vi "Main.vi"() -> ()   [LabVIEW 2014, in "Chart Module.lvlib"]
uses:
  Chart Module.lvlib
  Module Data--cluster.ctl
  Limits Argument--cluster.ctl
  <vilib>/Delacor/Delacor QMH/Libraries/Message Queue_class/Delacor_lib_QMH_Message Queue.lvclass/Delacor_lib_QMH_Message Queue.ctl
  Send Value Argument--cluster.ctl
  Show Panel Argument--cluster.ctl
  Position--enum.ctl
  Stop Argument--cluster.ctl
  <vilib>/Delacor/Delacor QMH/Libraries/Message Queue_class/Delacor_lib_QMH_Enqueue Message (Single).vi
  <vilib>/Delacor/Delacor QMH/Libraries/Message Queue_class/Delacor_lib_QMH_Message Queue.lvclass
panel:
  in  "Title":bool
  out "Chart":T1(graph)
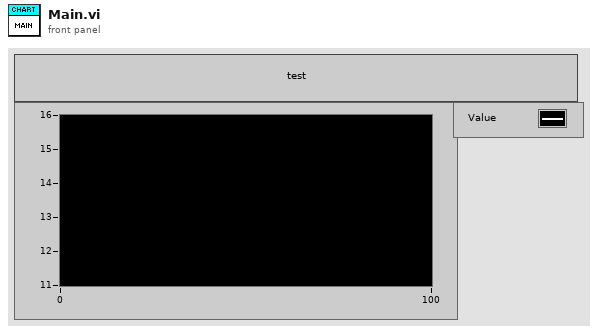
[diagram p1: front panel]
types:
  T1 = cluster{"Value":dbl, "HighLim":dbl, "LowLim":dbl}
  T2 = typedef "Chart Module.lvlib/Request Events--cluster.ctl" = cluster{"Stop Module":refnum<user-event>, "Show Panel":refnum<user-event>, "Hide Panel":refnum<user-event>, "Update Limits":refnum<user-event>, "Send Value":refnum<user-event>, "Clear Chart":refnum<user-event>, "Show Block Diagram":refnum<user-event>}
  T3 = typedef "Chart Module.lvlib/Module Data--cluster.ctl" = cluster{"Status":string, "Limits ":T4}
  T4 = typedef "Chart Module.lvlib/Limits Argument--cluster.ctl" = cluster{"Enabled?":bool, "HighLim":dbl, "LowLim":dbl}
  T5 = typedef "Chart Module.lvlib/Stop Argument--cluster.ctl" = cluster{"Origin":string, "Exit via Stop Module Req?":bool}
  T6 = typedef "Chart Module.lvlib/Show Panel Argument--cluster.ctl" = cluster{"Show Chart?":bool, "Chart Title":string, "Window Position":T7}
  T7 = typedef "Chart Module.lvlib/Position--enum.ctl" = enum16{"Upper-Left", "Upper-Center", "Upper-Right", "Center-left", "Center", "Center-Right", "Bottom-Left", "Bottom-Center", "Bottom-Right", ""}
  T8 = typedef "Chart Module.lvlib/Send Value Argument--cluster.ctl" = cluster{"Value":dbl}
  T9 = cluster{"Shift":bool, "Ctrl":bool, "Alt":bool, "Cmd":bool, "Opt":bool}
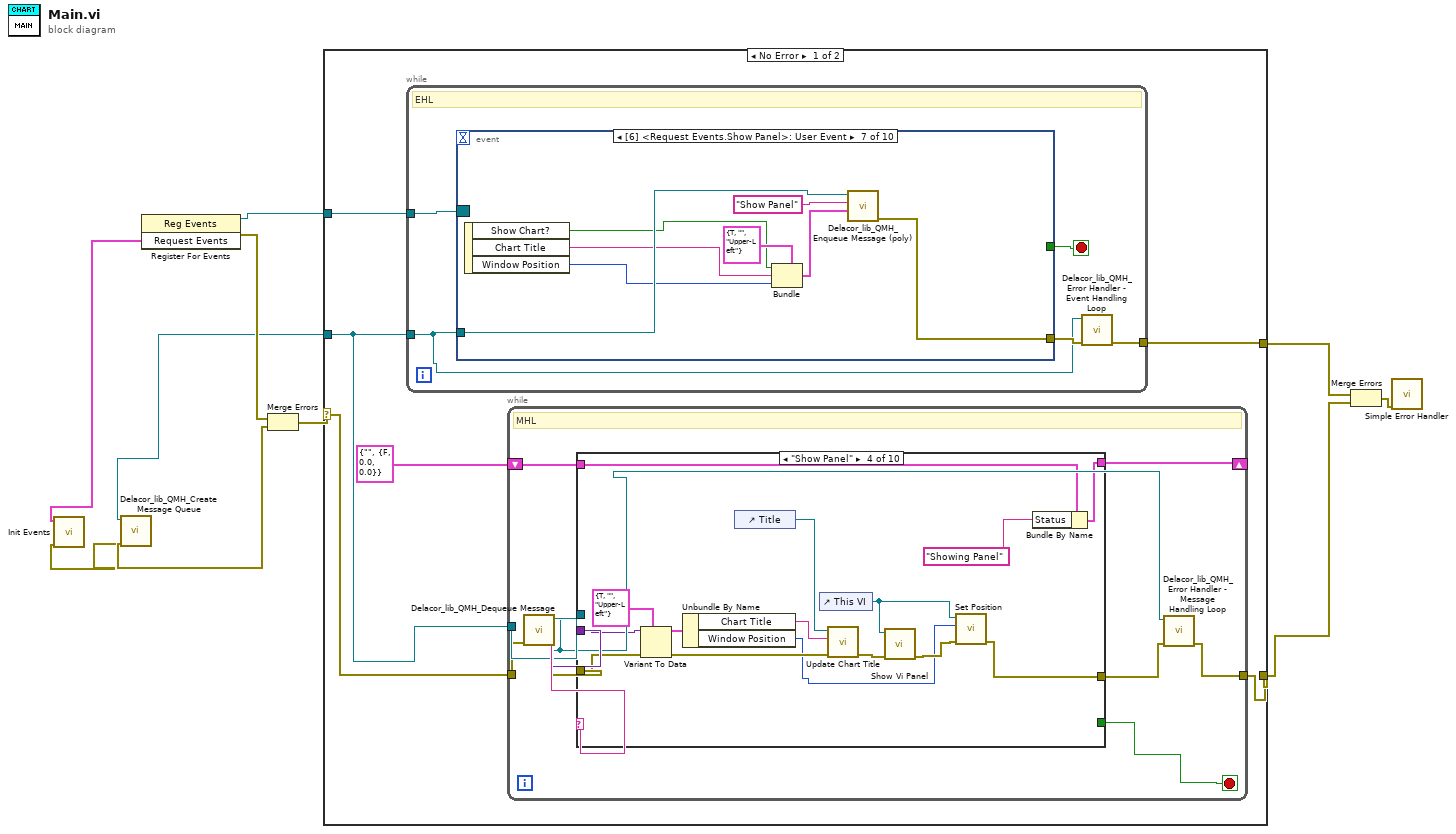
[diagram p0: block diagram]
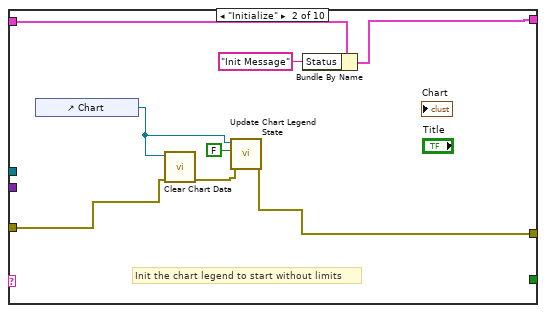
[diagram p3: hidden frame]
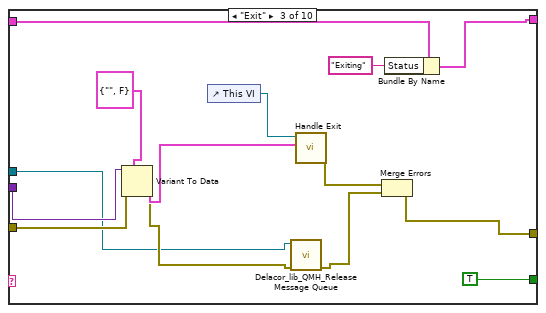
[diagram p4: hidden frame]
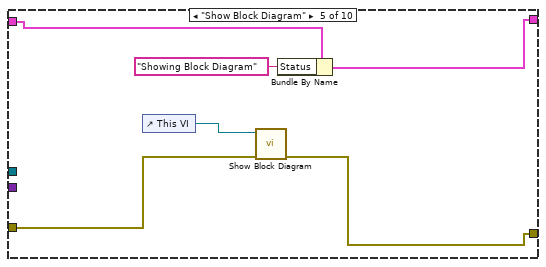
[diagram p5: hidden frame]
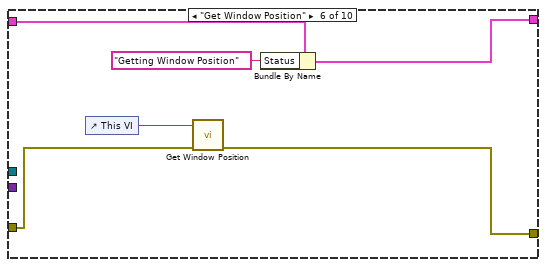
[diagram p6: hidden frame]
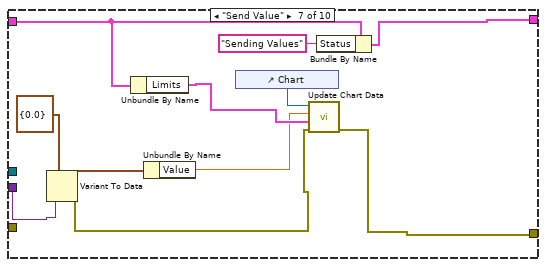
[diagram p7: hidden frame]
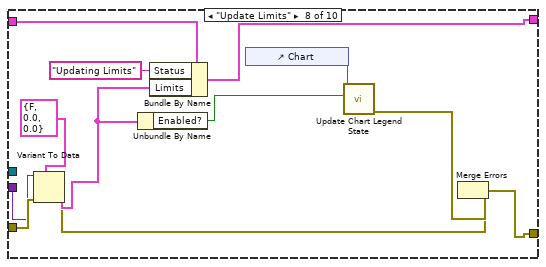
[diagram p8: hidden frame]
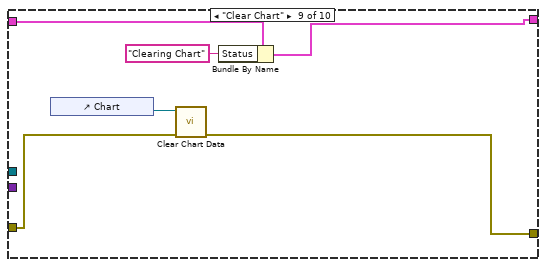
[diagram p9: hidden frame]
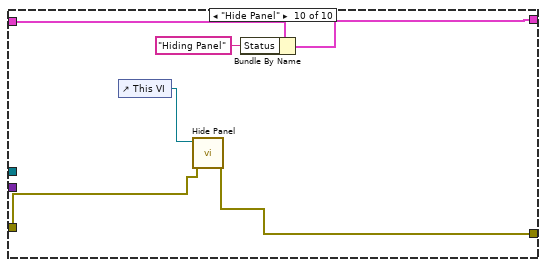
[diagram p10: hidden frame]
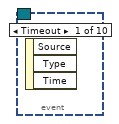
[diagram p11: hidden frame]
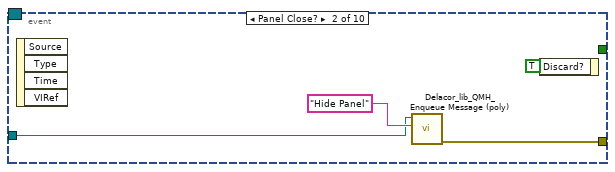
[diagram p12: hidden frame]
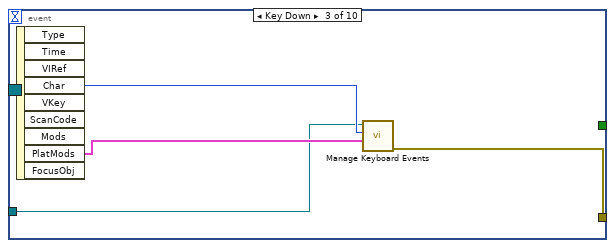
[diagram p13: hidden frame]
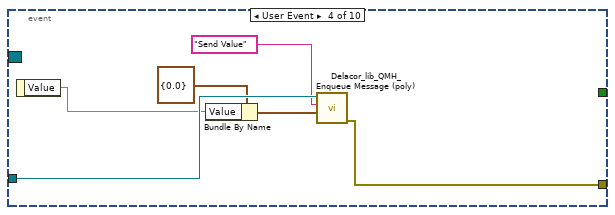
[diagram p14: hidden frame]
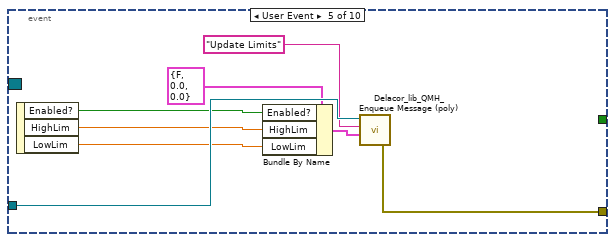
[diagram p15: hidden frame]
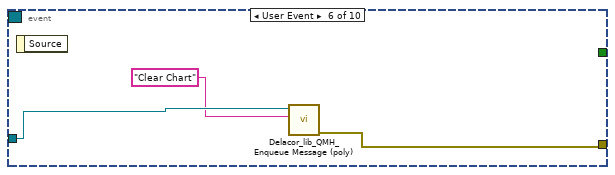
[diagram p16: hidden frame]
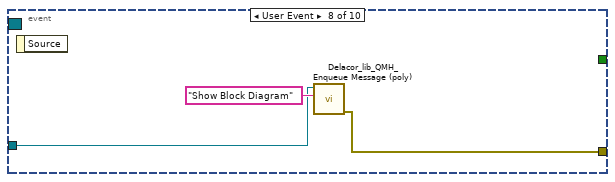
[diagram p17: hidden frame]
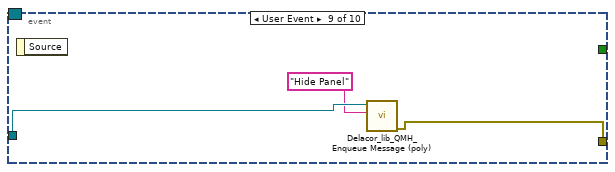
[diagram p18: hidden frame]
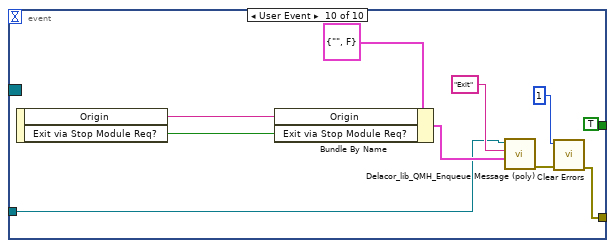
[diagram p19: hidden frame]
diagram:
  n1 = call "Init Events.vi"() -> ("error out"=w5:errorcluster, "Request Events"=w6:T2)  [unwired: 10 in]
  n2 = call <vilib>:"Delacor_lib_QMH_Create Message Queue.vi"("error in"=w5) -> ("error out"=w7:errorcluster, "Message Queue"=w4:refnum<class "Delacor_lib_QMH_Message Queue.lvclass">)  [unwired: 9 in]
  n3 = register-events(w6) -> (reference out=w8:refnum<event-registration>, error out=w9:errorcluster)  [unwired: 2 in]
  n4 = Merge Errors(w9, w7) -> (w10:errorcluster)
  n5 = case shown="No Error" w10 {
    selector: w10 -> [w11 _]
    tunnel: w8 -> [w16 _]
    tunnel: w4 -> [w15 _]
    tunnel: [w14 _] -> w3
    tunnel: [w13 _] -> w2
    frame No Error {
      n6 = while {
        tunnel: w16 -> [w118]
        tunnel: w15 -> [w114]
        tunnel: [w116] -> w14
        stop <- w115 stop-if-true
        # "EHL"
        n7 = event shown="[6] <Request Events.Show Panel>: User Event" {
          selector: w118 -> [_ _ _ _ _ _ _ _ _ _]
          dyn-events: _ -> [_ _ _ _ _ _ _ _ _ _]
          timeout: _ -> [_ _ _ _ _ _ _ _ _ _]
          tunnel: w114 -> [_ w121 w124 w132 w140 w143 w151 w152 w157 w162]
          tunnel: [_ w120 w123 w130 w133 w141 w149 w153 w155 w159] -> w117
          tunnel: [_ _ _ _ _ _ _ _ _ TRUE] -> w115
          event Timeout {
            n8 = event-data() -> ()  [unwired: 1 in, 3 out]
          }
          event Panel Close? {
            n9 = event-data() -> ()  [unwired: 1 in, 4 out]
            n10 = call-poly <vilib>:"Delacor_lib_QMH_Enqueue Message (poly).vi"("Message"="Hide Panel", "Message Queue in"=w121) -> ("error out"=w120:errorcluster)  [unwired: 8 in, 1 out]
            n11 = event-data("Discard?"=TRUE) -> ()  [unwired: 1 in, 1 out]
          }
          event Key Down {
            n12 = event-data() -> ("Char"=w125:i16, "PlatMods"=w126:T9)  [unwired: 1 in, 7 out]
            n13 = call "Manage Keyboard Events.vi"("PlatMods"=w126, "Char"=w125, "Delacor_lib_QMH_Message Queue in"=w124) -> ("error out"=w123:errorcluster)  [unwired: 8 in]
          }
          event User Event {
            n14 = event-data() -> ("Value"=w128:dbl)  [unwired: 1 in]
            n15 = Bundle By Name(cluster=T8 {"Value"=0.0} ("Send Value Argument"), "Value"=w128) -> (w127:T8)
            n16 = call-poly <vilib>:"Delacor_lib_QMH_Enqueue Message (poly).vi"("Message Data"=w127, "Message"="Send Value", "Message Queue in"=w132) -> ("error out"=w130:errorcluster)  [unwired: 7 in, 1 out]
          }
          event User Event {
            n17 = event-data() -> ("Enabled?"=w135:bool, "HighLim"=w136:dbl, "LowLim"=w137:dbl)  [unwired: 1 in]
            n18 = Bundle By Name(cluster=T4 {"Enabled?"=FALSE, "HighLim"=0.0, "LowLim"=0.0} ("Limits Argument"), "Enabled?"=w135, "HighLim"=w136, "LowLim"=w137) -> (w134:T4)
            n19 = call-poly <vilib>:"Delacor_lib_QMH_Enqueue Message (poly).vi"("Message Data"=w134, "Message"="Update Limits", "Message Queue in"=w140) -> ("error out"=w133:errorcluster)  [unwired: 7 in, 1 out]
          }
          event User Event {
            n20 = event-data() -> ()  [unwired: 1 in, 1 out]
            n21 = call-poly <vilib>:"Delacor_lib_QMH_Enqueue Message (poly).vi"("Message"="Clear Chart", "Message Queue in"=w143) -> ("error out"=w141:errorcluster)  [unwired: 8 in, 1 out]
          }
          event User Event {
            n22 = event-data() -> ("Show Chart?"=w147:bool, "Chart Title"=w146:string, "Window Position"=w144:T7)  [unwired: 1 in]
            n23 = Bundle(cluster=T6 {"Show Chart?"=TRUE, "Chart Title"="", "Window Position"=enum."Upper-Left"} ("Show Panel Argument"), "Show Chart?"=w147, "Chart Title"=w146, "Window Position"=w144) -> (w145:T6)
            n24 = call-poly <vilib>:"Delacor_lib_QMH_Enqueue Message (poly).vi"("Message Data"=w145, "Message"="Show Panel", "Message Queue in"=w151) -> ("error out"=w149:errorcluster)  [unwired: 7 in, 1 out]
          }
          event User Event {
            n25 = event-data() -> ()  [unwired: 1 in, 1 out]
            n26 = call-poly <vilib>:"Delacor_lib_QMH_Enqueue Message (poly).vi"("Message"="Show Block Diagram", "Message Queue in"=w152) -> ("error out"=w153:errorcluster)  [unwired: 8 in, 1 out]
          }
          event User Event {
            n27 = event-data() -> ()  [unwired: 1 in, 1 out]
            n28 = call-poly <vilib>:"Delacor_lib_QMH_Enqueue Message (poly).vi"("Message"="Hide Panel", "Message Queue in"=w157) -> ("error out"=w155:errorcluster)  [unwired: 8 in, 1 out]
          }
          event User Event {
            n29 = event-data() -> ("Origin"=w167:string, "Exit via Stop Module Req?"=w166:bool)  [unwired: 1 in]
            n30 = Bundle By Name(cluster=T5 {"Origin"="", "Exit via Stop Module Req?"=FALSE} ("Stop Argument"), "Origin"=w167, "Exit via Stop Module Req?"=w166) -> (w164:T5)
            n31 = call-poly <vilib>:"Delacor_lib_QMH_Enqueue Message (poly).vi"("Message Data"=w164, "Message"="Exit", "Message Queue in"=w162) -> ("error out"=w160:errorcluster)  [unwired: 7 in, 1 out]
            n32 = call <vilib>:"Clear Errors.vi"("error in (no error)"=w160, "specific error code to clear (0: all)"=1) -> ("error out"=w159:errorcluster)  [unwired: 4 in, 1 out]
          }
        }
        n33 = call-dynamic "Delacor_lib_QMH_Error Handler - Event Handling Loop.vi"("error in"=w117, "Message Queue in"=w114) -> ("dup error in"=w116:errorcluster)  [unwired: 8 in, 1 out]
      }
      n34 = while {
        tunnel: w15 -> [w22]
        tunnel: [w24] -> w13
        shift-right: [w19] -> _
        shift-left: T3 {"Status"="", "Limits "={"Enabled?"=FALSE, "HighLim"=0.0, "LowLim"=0.0}} ("Module Data") -> [w20]
        tunnel: w11 -> [w18]
        stop <- w21 stop-if-true
        # "MHL"
        n35 = call-dynamic "Delacor_lib_QMH_Dequeue Message.vi"("error in"=w18, "Message Queue in"=w22) -> ("error out"=w25:errorcluster, "Message Data"=w26:variant, "Message"=w27:string, "Message Queue out"=w17:refnum<class "Delacor_lib_QMH_Message Queue.lvclass">)  [unwired: 6 in]
        n36 = case shown="\"Show Panel\"" w27 {
          tunnel: w17 -> [_ _ w43 _ _ _ _ _ _ _]
          tunnel: w26 -> [_ _ w50 w61 _ _ w89 w100 _ _]
          tunnel: w25 -> [w29 w34 w49 w63 w71 w75 _ w101 w107 w112]
          tunnel: [w29 w32 w44 w55 w70 w74 w81 w93 w106 w111] -> w23
          tunnel: [_ _ TRUE _ _ _ _ _ _ _] -> w21
          tunnel: w20 -> [w28 w37 w40 w66 w69 w77 w86 w98 w105 w110]
          tunnel: [w28 w36 w39 w65 w68 w78 w85 w97 w104 w109] -> w19
          frame "Def", Default {
          }
          frame "Initialize" {
            # "Init the chart legend to start without limits"
            n37 = control-ref of="Chart"() -> (w31:refnum<vi>)
            n38 = call "Clear Chart Data.vi"("error in (no error)"=w34, "WaveformChart in"=w31) -> ("error out"=w33:errorcluster)  [unwired: 9 in]
            n39 = call "Update Chart Legend State.vi"("error in"=w33, "Enabled?"=FALSE, "WaveformChart in"=w31) -> ("error out"=w32:errorcluster)  [unwired: 8 in]
            n40 = Bundle By Name(cluster=w37, "Status"="Init Message") -> (w36:T3)
          }
          frame "Exit" {
            n41 = Variant To Data(error in=w49, type=T5 {"Origin"="", "Exit via Stop Module Req?"=FALSE} ("Stop Argument"), Variant=w50) -> (data=w48:T5, error out=w47:errorcluster)
            n42 = control-ref of="This VI"() -> (w41:refnum<vi>)
            n43 = call-dynamic "Delacor_lib_QMH_Release Message Queue.vi"("error in"=w47, "Message Queue"=w43) -> ("error out"=w45:errorcluster)  [unwired: 9 in]
            n44 = call "Handle Exit.vi"("Stop Argument"=w48, "Vi Ref"=w41) -> ("error out"=w46:errorcluster)  [unwired: 9 in]
            n45 = Merge Errors(w46, w45) -> (w44:errorcluster)
            n46 = Bundle By Name(cluster=w40, "Status"="Exiting") -> (w39:T3)
          }
          frame "Show Panel" {
            n47 = Variant To Data(error in=w63, type=T6 {"Show Chart?"=TRUE, "Chart Title"="", "Window Position"=enum."Upper-Left"} ("Show Panel Argument"), Variant=w61) -> (data=w60:T6, error out=w58:errorcluster)
            n48 = Unbundle By Name(w60) -> ("Chart Title"=w59:string, "Window Position"=w52:T7)
            n49 = control-ref of="Title"() -> (w57:refnum<vi>)
            n50 = control-ref of="This VI"() -> (w53:refnum<vi>)
            n51 = call "Update Chart Title.vi"("error in (no error)"=w58, "Chart Title"=w59, "Boolean in"=w57) -> ("error out"=w56:errorcluster)  [unwired: 8 in]
            n52 = call "Show Vi Panel.vi"("error in (no error)"=w56, "Vi Ref"=w53) -> ("error out"=w54:errorcluster)  [unwired: 9 in]
            n53 = call "Set Position.vi"("error in (no error)"=w54, "Positions"=w52, "VI in"=w53) -> ("error out"=w55:errorcluster)  [unwired: 8 in]
            n54 = Bundle By Name(cluster=w66, "Status"="Showing Panel") -> (w65:T3)
          }
          frame "Show Block Diagram" {
            n55 = control-ref of="This VI"() -> (w72:refnum<vi>)
            n56 = call "Show Block Diagram.vi"("error in"=w71, "VI in"=w72) -> ("error out"=w70:errorcluster)  [unwired: 9 in]
            n57 = Bundle By Name(cluster=w69, "Status"="Showing Block Diagram") -> (w68:T3)
          }
          frame "Get Window Position" {
            n58 = control-ref of="This VI"() -> (w73:refnum<vi>)
            n59 = call "Get Window Position.vi"("error in (no error)"=w75, "VI in"=w73) -> ("error out"=w74:errorcluster)  [unwired: 9 in]
            n60 = Bundle By Name(cluster=w77, "Status"="Getting Window Position") -> (w78:T3)
          }
          frame "Send Value" {
            n61 = Variant To Data(type=T8 {"Value"=0.0} ("Send Value Argument"), Variant=w89) -> (data=w87:T8, error out=w80:errorcluster)  [unwired: 1 in]
            n62 = Unbundle By Name(w86) -> ("Limits"=w82:T4)
            n63 = Unbundle By Name(w87) -> ("Value"=w79:dbl)
            n64 = control-ref of="Chart"() -> (w83:refnum<vi>)
            n65 = call "Update Chart Data.vi"("error in (no error)"=w80, "Limits"=w82, "Value"=w79, "WaveformChart in"=w83) -> ("error out"=w81:errorcluster)  [unwired: 7 in]
            n66 = Bundle By Name(cluster=w86, "Status"="Sending Values") -> (w85:T3)
          }
          frame "Update Limits" {
            n67 = Variant To Data(error in=w101, type=T4 {"Enabled?"=FALSE, "HighLim"=0.0, "LowLim"=0.0} ("Limits Argument"), Variant=w100) -> (data=w95:T4, error out=w91:errorcluster)
            n68 = Unbundle By Name(w95) -> ("Enabled?"=w94:bool)
            n69 = Bundle By Name(cluster=w98, "Status"="Updating Limits", "Limits"=w95) -> (w97:T3)
            n70 = control-ref of="Chart"() -> (w90:refnum<vi>)
            n71 = call "Update Chart Legend State.vi"("Enabled?"=w94, "WaveformChart in"=w90) -> ("error out"=w92:errorcluster)  [unwired: 9 in]
            n72 = Merge Errors(w92, w91) -> (w93:errorcluster)
          }
          frame "Clear Chart" {
            n73 = control-ref of="Chart"() -> (w102:refnum<vi>)
            n74 = call "Clear Chart Data.vi"("error in (no error)"=w107, "WaveformChart in"=w102) -> ("error out"=w106:errorcluster)  [unwired: 9 in]
            n75 = Bundle By Name(cluster=w105, "Status"="Clearing Chart") -> (w104:T3)
          }
          frame "Hide Panel" {
            n76 = control-ref of="This VI"() -> (w113:refnum<vi>)
            n77 = call "Hide Panel.vi"("error in (no error)"=w112, "Vi Ref"=w113) -> ("error out"=w111:errorcluster)  [unwired: 9 in]
            n78 = Bundle By Name(cluster=w110, "Status"="Hiding Panel") -> (w109:T3)
          }
        }
        n79 = call-dynamic "Delacor_lib_QMH_Error Handler - Message Handling Loop.vi"("error in"=w23, "Message Queue in"=w17) -> ("dup error in"=w24:errorcluster)  [unwired: 8 in, 1 out]
      }
    }
    frame Error {
    }
  }
  n80 = Merge Errors(w3, w2) -> (w1:errorcluster)
  n81 = call <vilib>:"Simple Error Handler.vi"("error in (no error)"=w1) -> ()  [unwired: 4 in, 5 out]
